vi "Timer z zajec.vi"(10 "T start/ F stop":bool) -> (2 "Time ms":u32)   [LabVIEW 2013]
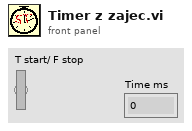
[diagram p1: front panel]
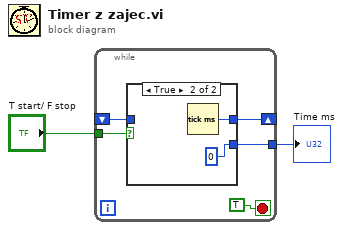
[diagram p0: block diagram]
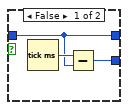
[diagram p2: hidden frame]
diagram:
  n1 = while {
    shift-right: [w5] -> _
    shift-left: _ -> [w4]
    tunnel: "T start/ F stop" -> [w6]
    tunnel: [w3] -> w1
    stop <- TRUE stop-if-true
    n2 = case shown="True" w6 {
      tunnel: [w8 w12] -> w5
      tunnel: w4 -> [w8 _]
      tunnel: [w9 u32 0] -> w3
      frame False {
        n3 = Tick Count (ms)() -> (millisecond timer value=w10:u32)
        n4 = Subtract(x=w10, y=w8) -> (x-y=w9:u32)
      }
      frame True {
        n5 = Tick Count (ms)() -> (millisecond timer value=w12:u32)
      }
    }
  }
  "Time ms" <- w1
